vi "Test_ValueReferenceTransport_ValueOK.vi"(8 "error in (no error)":errorcluster, 11 "TestCase in":refnum<class "TestTransport.lvclass">) -> (0 "error out":errorcluster, 3 "TestCase out":refnum<class "TestTransport.lvclass">)   [LabVIEW 2017, in "TestTransport.lvclass"]
uses:
  TestTransport.lvclass
  ValueReferenceTransport/ValueReferenceTransport.lvclass/ValueReferenceTransport.ctl
  <vilib>/Utility/error.llb/Error Cluster From Error Code.vi
  ValueReferenceTransport/ValueReferenceTransport.lvclass
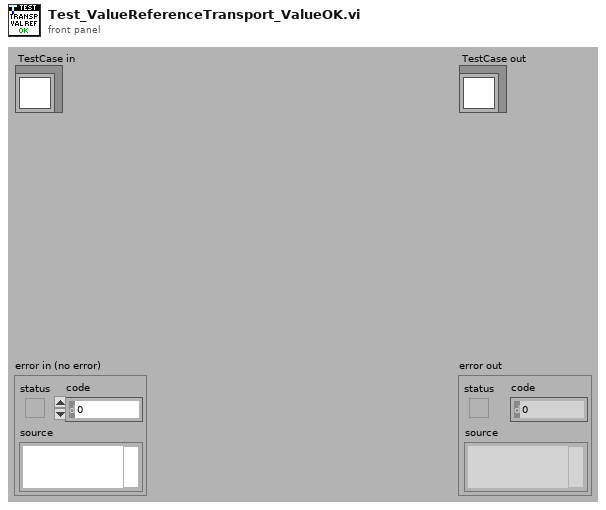
[diagram p1: front panel]
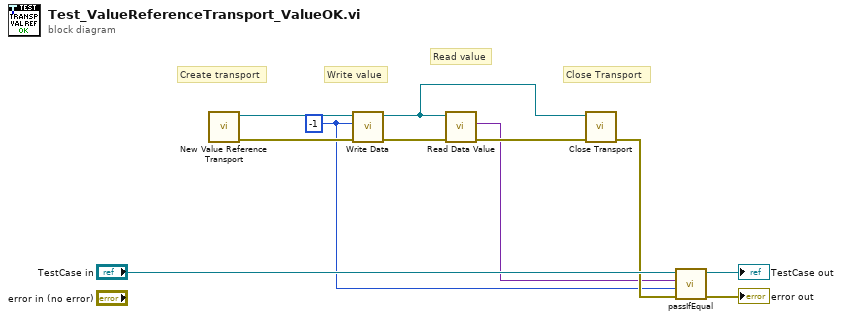
[diagram p0: block diagram]
diagram:
  w1 = -1
  # "Close Transport"
  # "Create transport"
  # "Write value"
  # "Read value"
  n1 = call "New Value Reference Transport.vi"() -> ("error out"=w7:errorcluster, "ValueReferenceTransport"=w8:refnum<class "ValueReferenceTransport.lvclass">)  [unwired: 10 in]
  n2 = call-dynamic "Write Data.vi"("error in (no error)"=w7, "Value"=w1, "ValueReferenceTransport In"=w8) -> ("error out"=w6:errorcluster, "ValueReferenceTransport Out"=w3:refnum<class "ValueReferenceTransport.lvclass">)  [unwired: 7 in]
  n3 = call "Read Data Value.vi"("error in (no error)"=w6, "ValueReferenceTransport In"=w3) -> ("error out"=w5:errorcluster, "Data"=w2:variant)  [unwired: 7 in, 1 out]
  n4 = call-dynamic "Close Transport.vi"("error in (no error)"=w5, "ValueReferenceTransport in"=w3) -> ("error out"=w4:errorcluster)  [unwired: 9 in]
  n5 = call-dynamic "passIfEqual.vi"("error in (no error)"=w4, "y"=w1, "x"=w2, "TestCase in"="TestCase in") -> ("error out"=→"error out":errorcluster, "TestCase out"=→"TestCase out":refnum<class "TestTransport.lvclass">)  [unwired: 6 in]
